vi "Unflatten Existing Configurations Test.vi"() -> (0 "Error Out":errorcluster, 2 "Pass":bool)   [LabVIEW 2014, in "Modbus Tests.lvlib"]
doc: "Test to make sure we can unflatten existing configurations correctly.\n\nUnlike the serialization test which creates a configuration object to flatten and then unflatten, we take a saved configuration string and unflatten it to make sure we can correctly read any existing configurations people are using."
uses:
  Modbus Tests.lvlib
  module/configuration/Modbus Module configuration.lvclass
  module/configuration/modbus class.ctl
  module/module channel/data bank type.ctl
  <vilib>/NI/Tag Bus Module Framework/channel/channel classification.ctl
  module/configuration/Modbus Module configuration.lvclass/Modbus Module configuration.ctl
  module/module channel/Modbus Module Channel.lvclass/Modbus Module Channel.ctl
  <vilib>/NI/Tag Bus Module Framework/channel/TBM channel.lvclass/TBM channel.ctl
  module/module channel/Read modbus type.vi
  module/module channel/Read starting address.vi
  <vilib>/NI/Tag Bus Module Framework/channel/Read channel classification.vi
  module/configuration/Read 32-bit first word low.vi
  module/configuration/Read 64-bit first dword low.vi
  module/configuration/Read baud rate.vi
  module/configuration/Read class.vi
  module/configuration/Read flow control (none).vi
  module/configuration/Read IP address.vi
  module/configuration/Read parity (even).vi
  module/configuration/Read port (502).vi
  module/configuration/Read unit ID.vi
  module/configuration/Read serial type.vi
  module/configuration/Read modbus channels.vi
  module/configuration/read force wire mode.vi
  module/module channel/Modbus Module Channel.lvclass
  <vilib>/NI/Tag Bus Module Framework/channel/TBM channel.lvclass
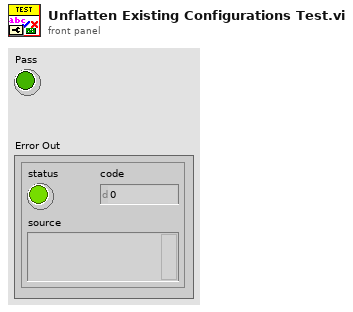
[diagram p1: front panel]
types:
  T1 = typedef "TBM channel.lvclass/channel classification.ctl" = enum16{"input data", "output data", "processing parameter", "processing result"}
  T2 = typedef "Modbus Module Channel.lvclass/data bank type.ctl" = enum16{"Coils", "Discrete Inputs", "Input Registers", "Holding Registers"}
  T3 = typedef "Modbus Module configuration.lvclass/modbus class.ctl" = enum16{"TCP master", "TCP slave", "serial master", "serial slave"}
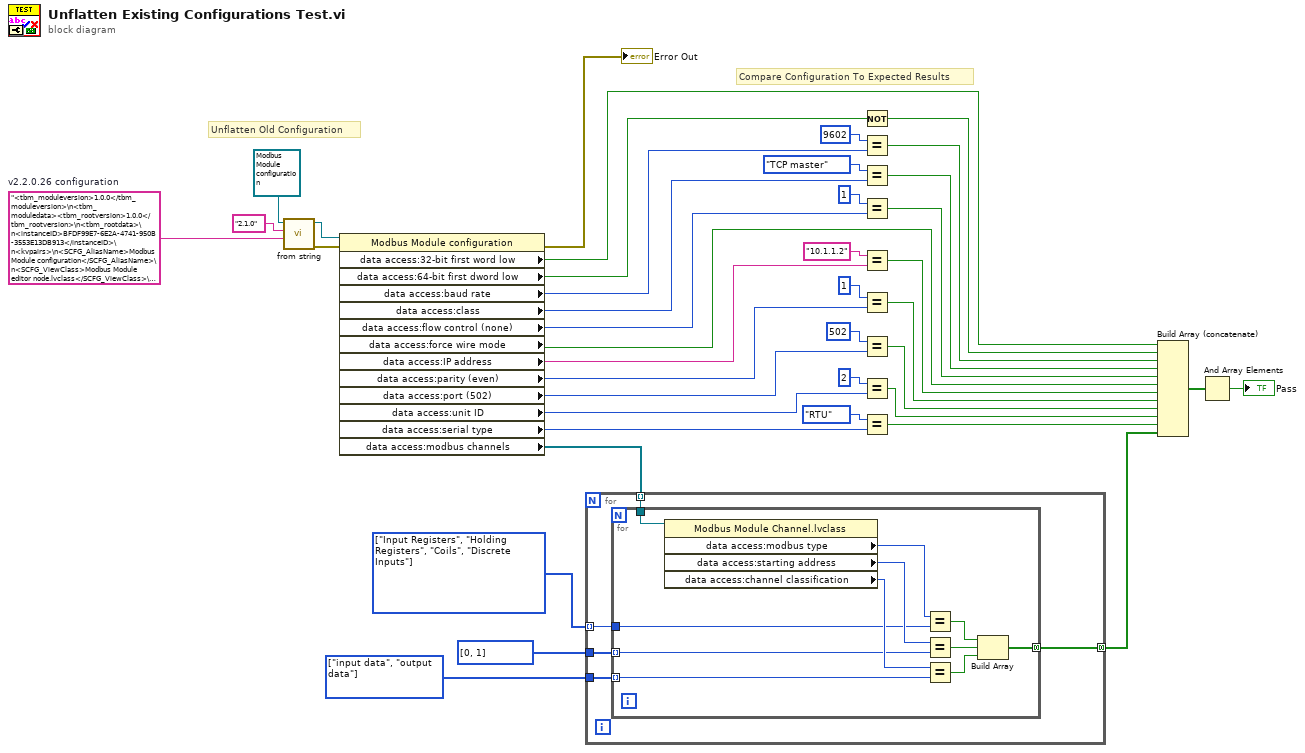
[diagram p0: block diagram]
diagram:
  w6 = T1[] [enum."input data", enum."output data"] items=["input data", "output data", "processing parameter", "processing result"]
  w8 = T2[] [enum."Input Registers", enum."Holding Registers", enum."Coils", enum."Discrete Inputs"] items=["Coils", "Discrete Inputs", "Input Registers", "Holding Registers"]
  w15 = "<tbm_moduleversion>1.0.0</tbm_moduleversion>\n<tbm_moduledata><tbm_rootversion>1.0.0</tbm_rootversion>\n<tbm_rootdata>\n<instanceID>BFDF99E7-6E2A-4741-950B-3553E13DB913</instanceID>\n<kvpairs>\n<SCFG_AliasName>Modbus Module configuration</SCFG_AliasName>\n<SCFG_ViewClass>Modbus Module editor node.lvclass</SCFG_ViewClass>\n</kvpairs>\n</tbm_rootdata></tbm_moduledata>\n<MBSlaveChannels><IR0><ch_class>input data</ch_class><default></default><meta></meta><ch_type>U16</ch_type><ch_version>1.0.0</ch_version><mbc_mbtype>input registers</mbc_mbtype><mbc_startaddr>0</mbc_startaddr><mbc_subindex>0</mbc_subindex></IR0>\n<IR1><ch_class>output data</ch_class><default></default><meta></meta><ch_type>U16</ch_type><ch_version>1.0.0</ch_version><mbc_mbtype>input registers</mbc_mbtype><mbc_startaddr>1</mbc_startaddr><mbc_subindex>0</mbc_subindex></IR1>\n<HR0><ch_class>input data</ch_class><default></default><meta></meta><ch_type>U16</ch_type><ch_version>1.0.0</ch_version><mbc_mbtype>holding registers</mbc_mbtype><mbc_startaddr>0</mbc_startaddr><mbc_subindex>0</mbc_subindex></HR0>\n<HR1><ch_class>output data</ch_class><default></default><meta></meta><ch_type>U16</ch_type><ch_version>1.0.0</ch_version><mbc_mbtype>holding registers</mbc_mbtype><mbc_startaddr>1</mbc_startaddr><mbc_subindex>0</mbc_subindex></HR1>\n<C0><ch_class>input data</ch_class><default></default><meta></meta><ch_type>Boolean</ch_type><ch_version>1.0.0</ch_version><mbc_mbtype>coils</mbc_mbtype><mbc_startaddr>0</mbc_startaddr><mbc_subindex>0</mbc_subindex></C0>\n<C1><ch_class>output data</ch_class><default></default><meta></meta><ch_type>Boolean</ch_type><ch_version>1.0.0</ch_version><mbc_mbtype>coils</mbc_mbtype><mbc_startaddr>1</mbc_startaddr><mbc_subindex>0</mbc_subindex></C1>\n<DI0><ch_class>input data</ch_class><default></default><meta></meta><ch_type>Boolean</ch_type><ch_version>1.0.0</ch_version><mbc_mbtype>discrete inputs</mbc_mbtype><mbc_startaddr>0</mbc_startaddr><mbc_subindex>0</mbc_subindex></DI0>\n<DI1><ch_class>output data</ch_class><default></default><meta></meta><ch_type>Boolean</ch_type><ch_version>1.0.0</ch_version><mbc_mbtype>discrete inputs</mbc_mbtype><mbc_startaddr>1</mbc_startaddr><mbc_subindex>0</mbc_subindex></DI1>\n</MBSlaveChannels>\n<MBSlavePort>502</MBSlavePort>\n<MBFlowCtl>1</MBFlowCtl>\n<MBSerADU>RTU</MBSerADU>\n<MBParity>1</MBParity>\n<MBUnitID>2</MBUnitID>\n<MBBaudRate>9602</MBBaudRate>\n<MBVisaResource></MBVisaResource>\n<MBClass>TCP master</MBClass>\n<MBTCPAddr>10.1.1.2</MBTCPAddr>\n<MBSERForceWireMode>TRUE</MBSERForceWireMode>\n<MBSERWireMode>0</MBSERWireMode><MBFirstWordLow>TRUE</MBFirstWordLow><MBFirstDWordLow>TRUE</MBFirstDWordLow>\n"  # v2.2.0.26 configuration
  # "Compare Configuration To Expected Results"
  # "Unflatten Old Configuration"
  n1 = call-dynamic "from string.vi"("data"=w15, "version"="2.1.0", "Modbus Slave configuration in"=refnum<class "Modbus Module configuration.lvclass"> refnum) -> ("error out"=w39:errorcluster, "Modbus Slave configuration out"=w40:refnum<class "Modbus Module configuration.lvclass">)  [unwired: 7 in]
  n2 = property class="Modbus Module configuration"(reference=w40, error in=w39) -> (error out=→"Error Out":errorcluster, "data access:32-bit first word low"=w38:bool, "data access:64-bit first dword low"=w37:bool, "data access:baud rate"=w35:u32, "data access:class"=w31:T3, "data access:flow control (none)"=w29:u16, "data access:force wire mode"=w13:bool, "data access:IP address"=w12:string, "data access:parity (even)"=w23:u16, "data access:port (502)"=w21:u16, "data access:unit ID"=w19:u8, "data access:serial type"=w16:enum16{"RTU", "ASCII"}, "data access:modbus channels"=w4:refnum<class "Modbus Module Channel.lvclass">[])  [unwired: 1 out]
  n3 = for {
    tunnel: w8 -> [w46] mode=indexing
    tunnel: u16[] [0, 1] -> [w45]
    tunnel: w6 -> [w44]
    tunnel: w4 -> [w43] mode=indexing
    tunnel: [w42] -> w3 mode=concatenating
    n4 = for {
      tunnel: w46 -> [w53]
      tunnel: w45 -> [w52] mode=indexing
      tunnel: w44 -> [w51] mode=indexing
      tunnel: w43 -> [w57]
      tunnel: [w47] -> w42 mode=concatenating
      n5 = property class="Modbus Module Channel.lvclass"(reference=w57) -> ("data access:modbus type"=w56:T2, "data access:starting address"=w55:u16, "data access:channel classification"=w54:T1)  [unwired: 1 in, 2 out]
      n6 = Equal?(x=w56, y=w53) -> (x = y?=w50:bool)
      n7 = Equal?(x=w55, y=w52) -> (x = y?=w49:bool)
      n8 = Equal?(x=w54, y=w51) -> (x = y?=w48:bool)
      n9 = Build Array(w50, w49, w48) -> (w47:bool[])
    }
  }
  n10 = Not(x=w37) -> (.not. x?=w36:bool)
  n11 = Equal?(x=u32 9602 ("baud rate"), y=w35) -> (x = y?=w33:bool)
  n12 = Equal?(x=modbus_class."TCP master" ("class"), y=w31) -> (x = y?=w30:bool)
  n13 = Equal?(x=u16 1 ("flow control (none)"), y=w29) -> (x = y?=w27:bool)
  n14 = Equal?(x="10.1.1.2", y=w12) -> (x = y?=w26:bool)
  n15 = Equal?(x=u16 1 ("parity (even)"), y=w23) -> (x = y?=w22:bool)
  n16 = Equal?(x=u16 502 ("parity (even)"), y=w21) -> (x = y?=w11:bool)
  n17 = Equal?(x=u16 2 ("parity (even)"), y=w19) -> (x = y?=w10:bool)
  n18 = Equal?(x=enum16{"RTU", "ASCII"}."RTU" ("serial type"), y=w16) -> (x = y?=w9:bool)
  n19 = Build Array (concatenate)(w38, w36, w33, w30, w27, w13, w26, w22, w11, w10, w9, w3) -> (w2:bool[])
  n20 = And Array Elements(Boolean array=w2) -> (logical AND=→"Pass":bool)
